vi "Process Secondary Input.vi"(11 "Ship in":refnum<class "Ship.lvclass">) -> (2 "New Elements":refnum<class "Element.lvclass">[](array[class]), 3 "Ship out":refnum<class "Ship.lvclass">)   [LabVIEW 2021, in "Ship.lvclass"]
uses:
  Ship.lvclass
  Element/Element.lvclass
  Ship.lvclass/Ship.ctl
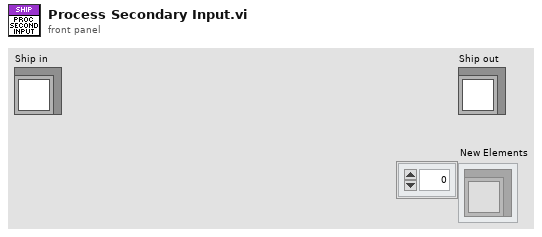
[diagram p1: front panel]
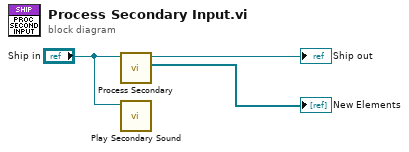
[diagram p0: block diagram]
diagram:
  n1 = call-dynamic "Process Secondary.vi"("Ship in"="Ship in") -> ("New Elements"=→"New Elements":refnum<class "Element.lvclass">[], "Ship out"=→"Ship out":refnum<class "Ship.lvclass">)  [unwired: 9 in]
  n2 = call-dynamic "Play Secondary Sound.vi"("Ship in"="Ship in") -> ()  [unwired: 9 in, 2 out]
